vi "change_objective.vi"(8 "error in (no error)":errorcluster, 10 "objectives":T1[](array[typedef]), 11 "objective":refnum<vi>) -> (0 "error out":errorcluster)   [LabVIEW 2010]
uses:
  common/clusters/plugin_specification.ctl
  components/ScanHead/GenericScanHead/GenericScanHead/trigger_enum.ctl
  components/Objective/GenericObjective/GenericObjective/GenericObjective.lvclass
  common/classes/GenericComponent/GenericComponent/GenericComponent.lvclass
  components/ScanHead/GenericScanHead/GenericScanHead/GenericScanHead.lvclass
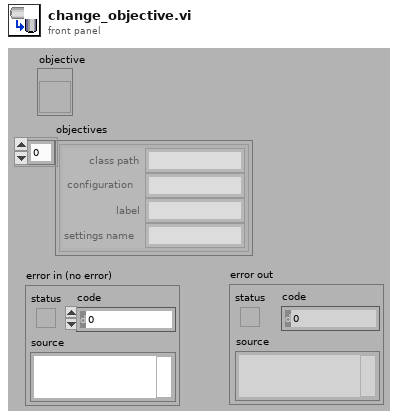
[diagram p1: front panel]
types:
  T1 = typedef "plugin_specification.ctl" = cluster{"class path":string, "configuration":string, "label":string, "settings name":string}
  T2 = typedef "GenericScanHead.lvclass/trigger_enum.ctl" = enum16{"NULL", "fetch trajectory", "generate trajectory", "change run mode", "update modifiers"}
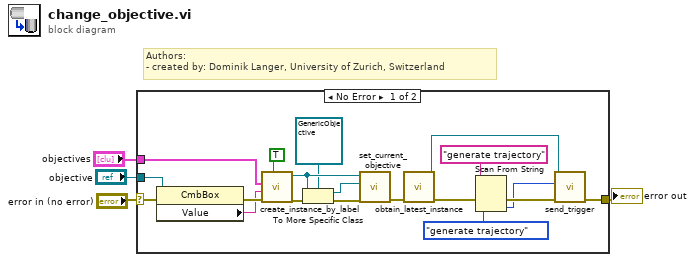
[diagram p0: block diagram]
diagram:
  # "Authors: \n- created by: Dominik Langer, University of Zurich, Switzerland"
  n1 = case shown="No Error" "error in (no error)" {
    selector: "error in (no error)" -> [w14 w24]
    tunnel: [w16 w24] -> w3
    tunnel: "objective" -> [w11 _]
    tunnel: "objectives" -> [w10 _]
    frame No Error {
      n2 = property class="CmbBox"(reference=w11, error in=w14) -> (error out=w13:errorcluster, "Value"=w12:string)  [unwired: 1 out]
      n3 = call "create_instance_by_label.vi"("call constructor?"=TRUE, "error in (no error)"=w13, "label"=w12, "configuration list"=w10) -> ("error out"=w23:errorcluster, "GenericPlugin out"=w21:refnum<class "GenericComponent.lvclass">)  [unwired: 6 out]
      n4 = To More Specific Class(target class=refnum<class "GenericObjective.lvclass"> refnum ("GenericObjective.lvclass"), reference=w21, error in=w23) -> (specific class reference=w20:refnum<class "GenericObjective.lvclass">, error out=w22:errorcluster)
      n5 = call-dynamic "set_current_objective.vi"("error in (no error)"=w22, "current objective"=w20, "GenericPlugin in"=w21) -> ("error out"=w19:errorcluster)  [unwired: 7 in, 1 out]
      n6 = call "obtain_latest_instance.vi"("error in (no error)"=w19) -> ("error out"=w9:errorcluster, "GenericScanHead out"=w18:refnum<class "GenericScanHead.lvclass">)  [unwired: 9 in]
      n7 = Scan From String(input string="generate trajectory", error in=w9, default 1=trigger_enum."generate trajectory" ("trigger")) -> (error out=w8:errorcluster, output 1=w5:T2)  [unwired: 2 in, 2 out]
      n8 = call-dynamic "send_trigger.vi"("error in (no error)"=w8, "trigger"=w5, "GenericScanHead in"=w18) -> ("error out"=w16:errorcluster)  [unwired: 7 in, 1 out]
    }
    frame Error {
    }
  }
  "error out" <- w3
